vi "User Access Level FGV Unit Test.vi"() -> ()   [LabVIEW 2012]
panel:
  in  "访问安全区域":bool
  out "错误输出":cluster{"状态":bool, "代码":i32, "源":string}
  in  "错误输入":cluster{"状态":bool, "代码":i32, "源":string}
  in  "当前用户":string
  in  "设置用户访问级别":bool
  in  "停止":bool
  # "1.  为当前用户设置访问级别。"
  # "2.  通过验证对话框消息，测试访问级别。"
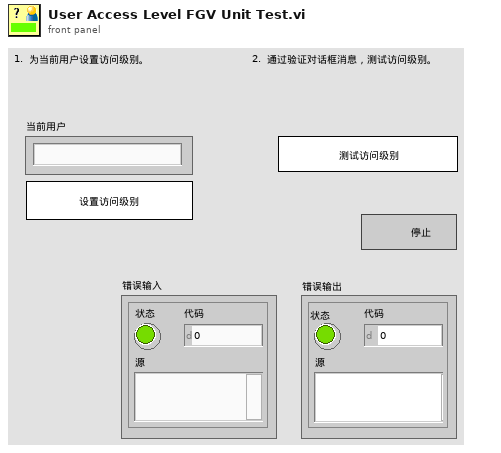
[diagram p1: front panel]
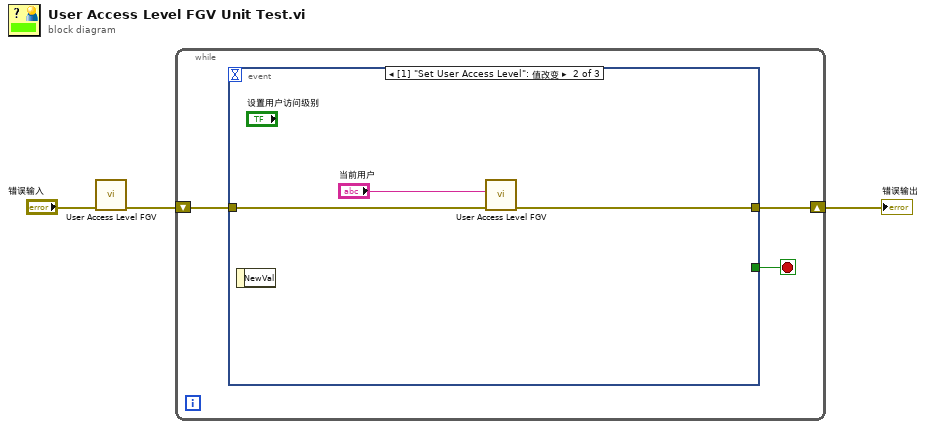
[diagram p0: block diagram]
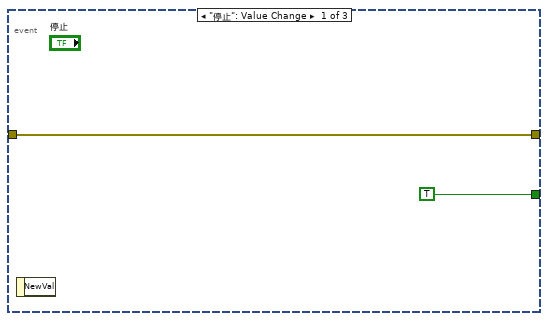
[diagram p2: hidden frame]
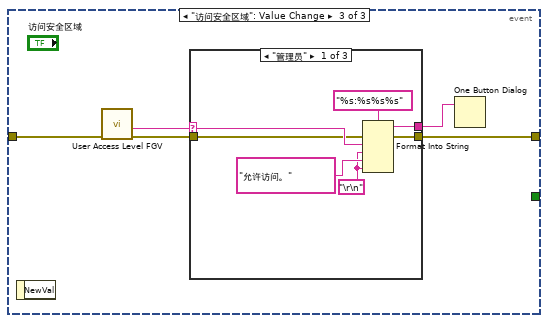
[diagram p3: hidden frame]
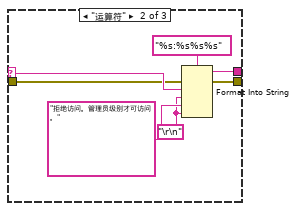
[diagram p4: hidden frame]
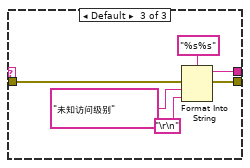
[diagram p5: hidden frame]
diagram:
  n1 = call "User Access Level FGV.vi"("错误输入"="错误输入") -> ("错误输出"=w3:cluster{"状态":bool, "代码":i32, "源":string})  [unwired: 9 in, 1 out]
  n2 = while {
    shift-right: [w4] -> w1
    shift-left: w3 -> [w5]
    stop <- w6 stop-if-true
    n3 = event shown="[1] \"Set User Access Level\": 值改变" {
      selector: _ -> [_ _ _]
      dyn-events: _ -> [_ _ _]
      timeout: _ -> [_ _ _]
      tunnel: [TRUE ("停止") _ _] -> w6
      tunnel: w5 -> [w7 w11 w16]
      tunnel: [w7 w9 w15] -> w4
      event "停止": Value Change {
        n4 = event-data ("事件数据节点")() -> ()  [unwired: 1 in, 1 out]
      }
      event "设置用户访问级别": Value Change {
        n5 = event-data ("事件数据节点")() -> ()  [unwired: 1 in, 1 out]
        n6 = call "User Access Level FGV.vi"("错误输入"=w11, "用户名"="当前用户") -> ("错误输出"=w9:cluster{"状态":bool, "代码":i32, "源":string})  [unwired: 8 in, 1 out]
      }
      event "访问安全区域": Value Change {
        n7 = event-data ("事件数据节点")() -> ()  [unwired: 1 in, 1 out]
        n8 = call "User Access Level FGV.vi"("错误输入"=w16) -> ("错误输出"=w14:cluster{"状态":bool, "代码":i32, "源":string}, "用户级别"=w13:string)  [unwired: 9 in]
        n9 = case shown="\"管理员\"" w13 {
          selector: w13 -> [w23 w30 _]
          tunnel: [w21 w28 w35] -> w15
          tunnel: w14 -> [w22 w29 w36]
          tunnel: [w17 w24 w33] -> w12
          frame "管理员" {
            w19 = "\r\n" ("行结束常量")
            n10 = Format Into String ("格式化写入字符串")(format string="%s:%s%s%s" ("格式字符串"), error in=w22, w23, w19, "允许访问。" ("消息"), w19) -> (resulting string=w17:string, error out=w21:errorcluster)  [unwired: 1 in]
          }
          frame "运算符" {
            w26 = "\r\n" ("行结束常量")
            n11 = Format Into String ("格式化写入字符串")(format string="%s:%s%s%s" ("格式字符串"), error in=w29, w30, w26, "拒绝访问。管理员级别才可访问。" ("消息"), w26) -> (resulting string=w24:string, error out=w28:errorcluster)  [unwired: 1 in]
          }
          frame Default {
            n12 = Format Into String ("格式化写入字符串")(format string="%s%s" ("格式字符串"), error in=w36, "未知访问级别" ("消息"), "\r\n" ("行结束常量")) -> (resulting string=w33:string, error out=w35:errorcluster)  [unwired: 1 in]
          }
        }
        n13 = One Button Dialog ("单按钮对话框")(message=w12) -> ()  [unwired: 1 in, 1 out]
      }
    }
  }
  "错误输出" <- w1
